vi "Set Mode (iSUB) (SubVI).vi"(5 "Mode":enum16{"Camera", "Video"}(ring)=enum."Video", 7 "REF IN":T1) -> ()   [LabVIEW 2015]
uses:
  <vilib>/rvi/interface/nirviReadWriteControl/nirviReadWriteControl.xnode
  Controls (HOST)/FPGA REF (iSUB).ctl
  NiFpgaLv.dll
  <vilib>/Utility/error.llb/Error Cluster From Error Code.vi
  <vilib>/rvi/interface/Simulation/niFpgaSimulationCallBeginRW.vi
  <vilib>/rvi/errors/niLvFpgaAdjustHostInterfaceError.vi
  Controls (HOST)/Data to Disk Bundle.ctl
  Controls (HOST)/Image Queue Bundle.ctl
  Controls (HOST)/REF.ctl
  Controls (HOST)/FPGA REF (MWT).ctl
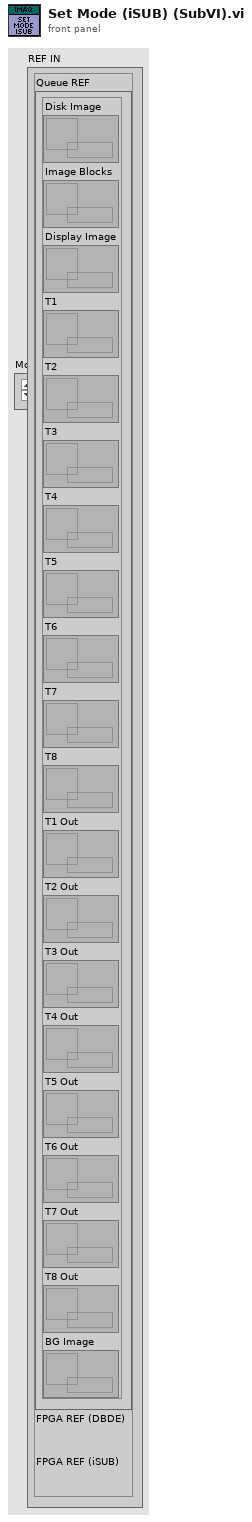
[diagram p1: front panel]
types:
  T1 = typedef "REF.ctl" = cluster{"Queue REF":T2, "FPGA REF (DBDE)":T3, "FPGA REF (iSUB)":T4}
  T2 = typedef "Image Queue Bundle.ctl" = cluster{"Disk Image":refnum<queue>, "Image Blocks":refnum<queue>, "Display Image":refnum<queue>, "T1":refnum<queue>, "T2":refnum<queue>, "T3":refnum<queue>, "T4":refnum<queue>, "T5":refnum<queue>, "T6":refnum<queue>, "T7":refnum<queue>, "T8":refnum<queue>, "T1 Out":refnum<queue>, "T2 Out":refnum<queue>, "T3 Out":refnum<queue>, "T4 Out":refnum<queue>, "T5 Out":refnum<queue>, "T6 Out":refnum<queue>, "T7 Out":refnum<queue>, "T8 Out":refnum<queue>, "BG Image":refnum<queue>}
  T3 = typedef "FPGA REF (MWT).ctl" = refnum<k20>
  T4 = typedef "FPGA REF (iSUB).ctl" = refnum<k20>
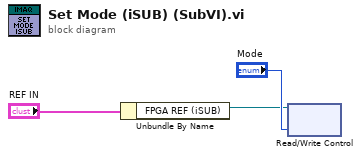
[diagram p0: block diagram]
diagram:
  n1 = Unbundle By Name("REF IN") -> ("FPGA REF (iSUB)"=w1:T4)
  n2 = xnode "Read/Write Control"("FPGA VI Reference In"=w1, "Mode"="Mode") -> ()  [unwired: 1 in, 2 out]
